vi "parse_package.vi"(8 "error in (no error)":errorcluster, 10 "Raw Package without Header":string, 11 "OXY_SCPI Reseource In":refnum<visa-resource-name>) -> (0 "error out":errorcluster, 2 "DataAllChannels":T1[](array[typedef]), 3 "OXY_SCPI Reseource Out":refnum<visa-resource-name>)   [LabVIEW 2020, in "OXYGEN_Datastream.lvlib"]
uses:
  OXYGEN_Datastream.lvlib
  TypeDefs/DataPoint_Variant.ctl
  TypeDefs/FGV_enum_GeneralInfo.ctl
panel:
  out "error pckg info":u32
  out "Error pckg size":u32
  out "error remeining string":string
  out "error pckg info":string
  out "Error pckg size":string
  out "substring before match":string
  out "packages array":string[](array[string])
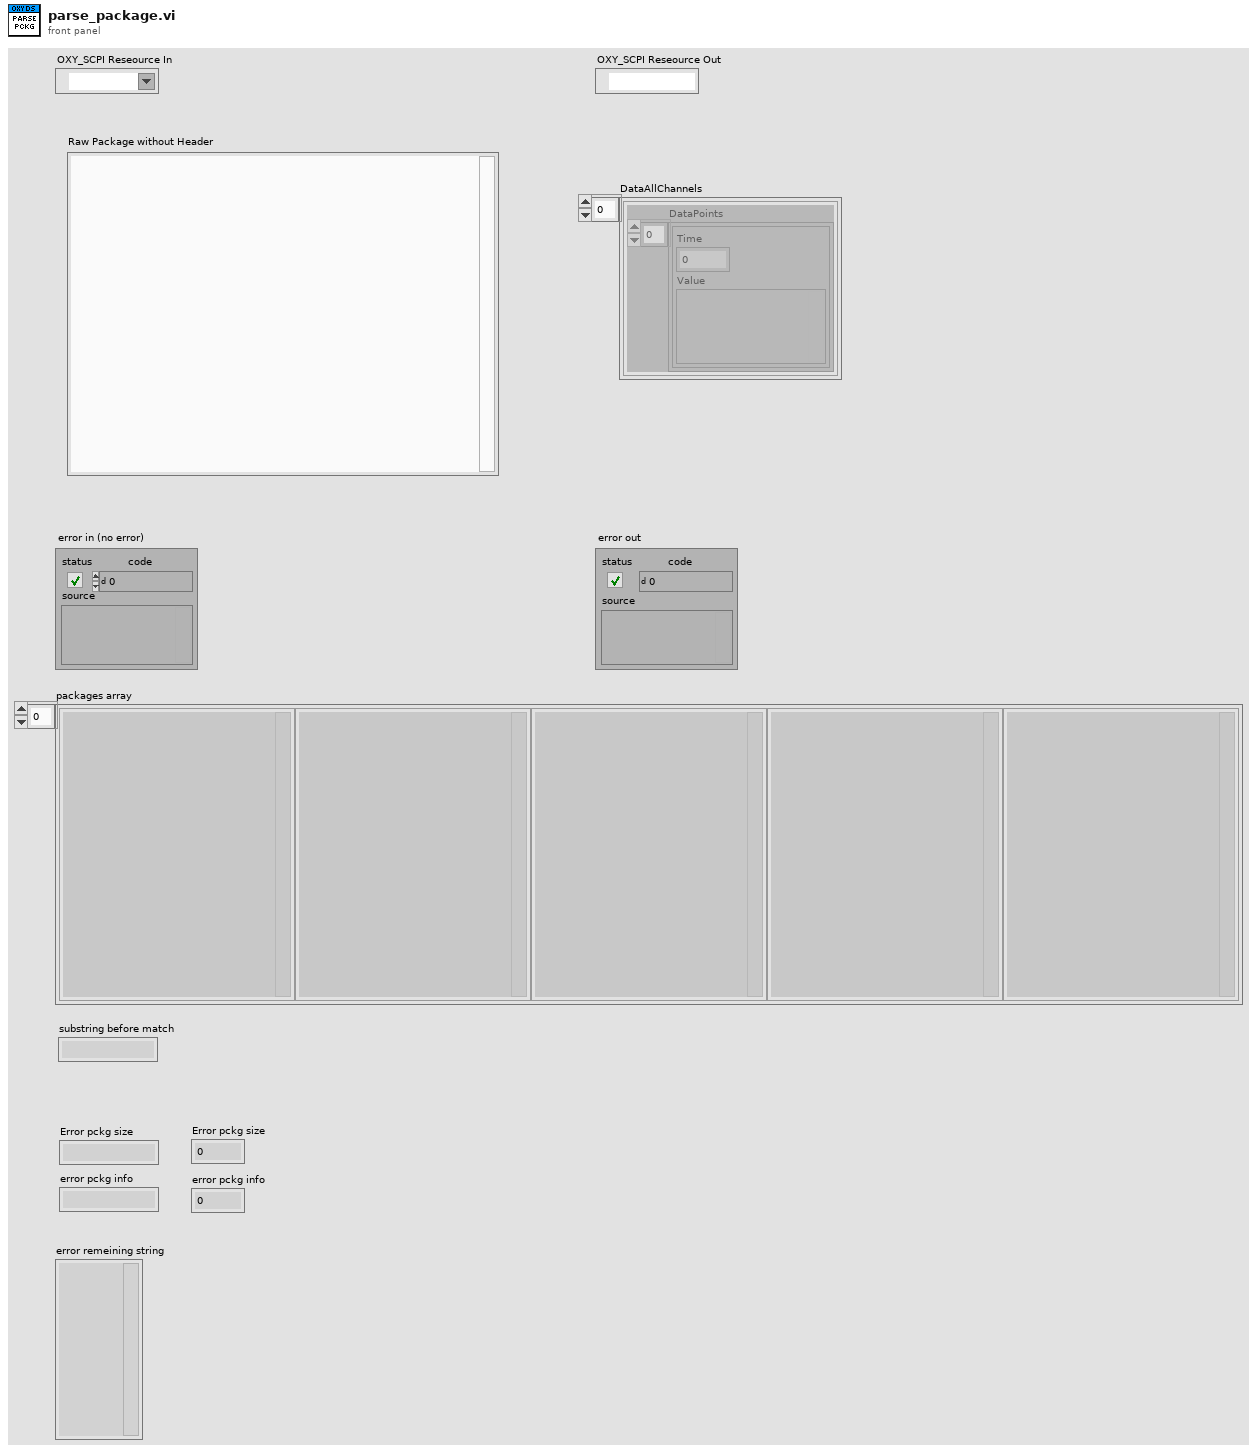
[diagram p1: front panel]
types:
  T1 = typedef "OXYGEN_Datastream.lvlib/DataPoint_Variant.ctl" = cluster{"DataPoints":cluster{"Time":dbl, "Value":variant}[]}
  T2 = typedef "OXYGEN_Datastream.lvlib/FGV_enum_GeneralInfo.ctl" = enum16{"Set_AcqInfo", "Set_ChInfo", "Get"}
  T3 = enum16{"big-endian, network order", "native, host order", "little-endian"}
  T4 = typedef "OXYGEN_Datastream.lvlib/ChannelInfo.ctl" = cluster{"Name":string, "Unit":string, "Scaling":T5}
  T5 = typedef "OXYGEN_Datastream.lvlib/ChannelInfo_Scaling.ctl" = cluster{"factor":dbl, "offset":dbl}
  T6 = typedef "OXYGEN_Datastream.lvlib/AcqInfo_AcquisitionStart.ctl" = cluster{"ISO8061":string, "nanoseconds":T7}
  T7 = typedef "OXYGEN_Datastream.lvlib/AcqInfo_AcquisitionStart_nanoseconds.ctl" = cluster{"utc_offset_seconds":i64, "timestamp_nanoseconds":i64}
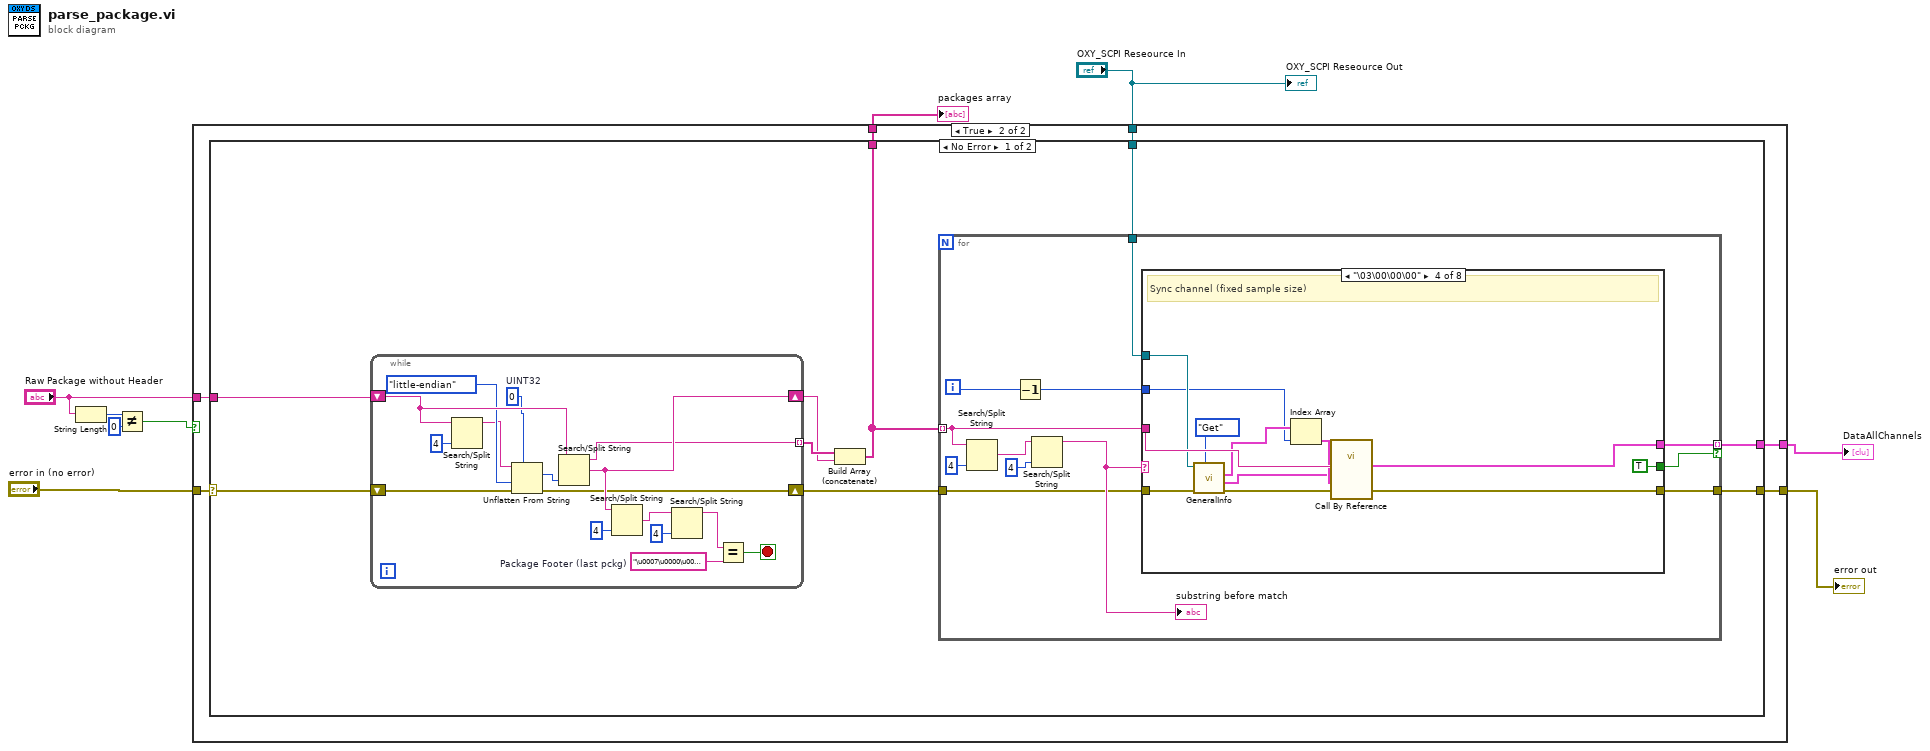
[diagram p0: block diagram]
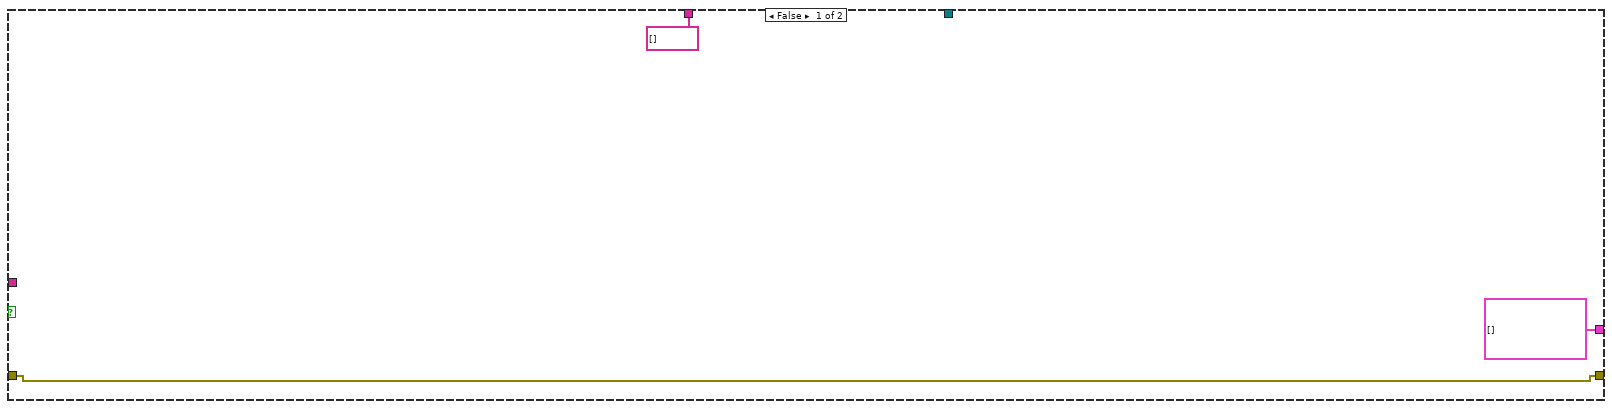
[diagram p2: hidden frame]
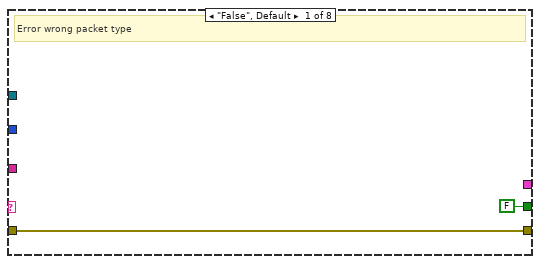
[diagram p3: hidden frame]
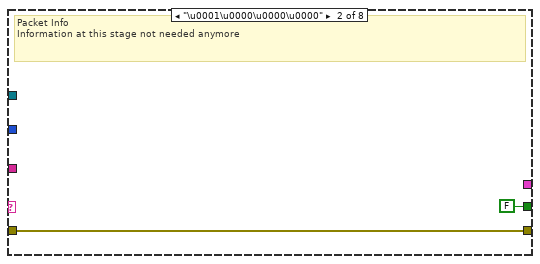
[diagram p4: hidden frame]
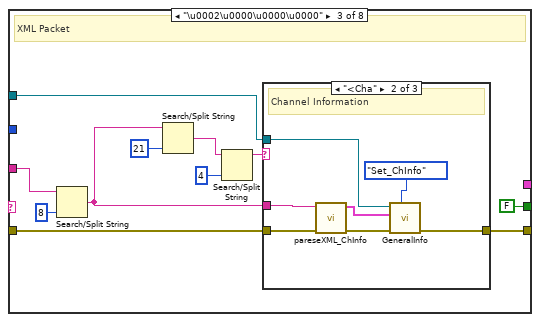
[diagram p5: hidden frame]
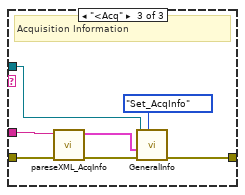
[diagram p7: hidden frame]
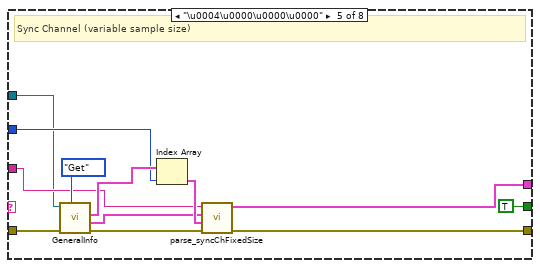
[diagram p8: hidden frame]
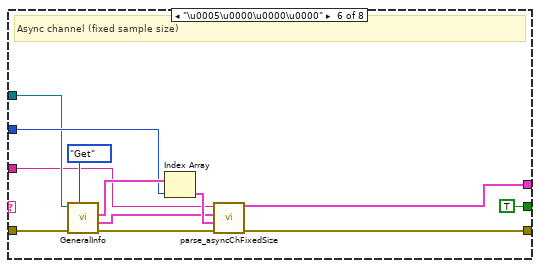
[diagram p9: hidden frame]
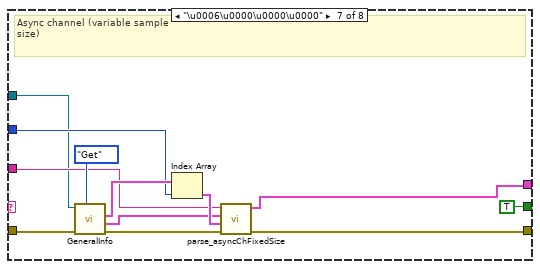
[diagram p10: hidden frame]
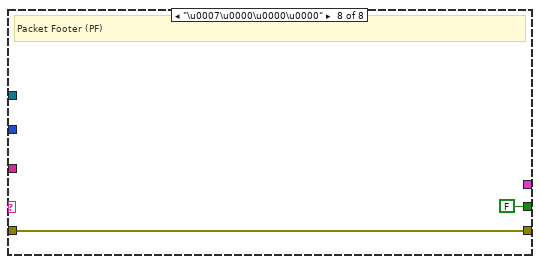
[diagram p11: hidden frame]
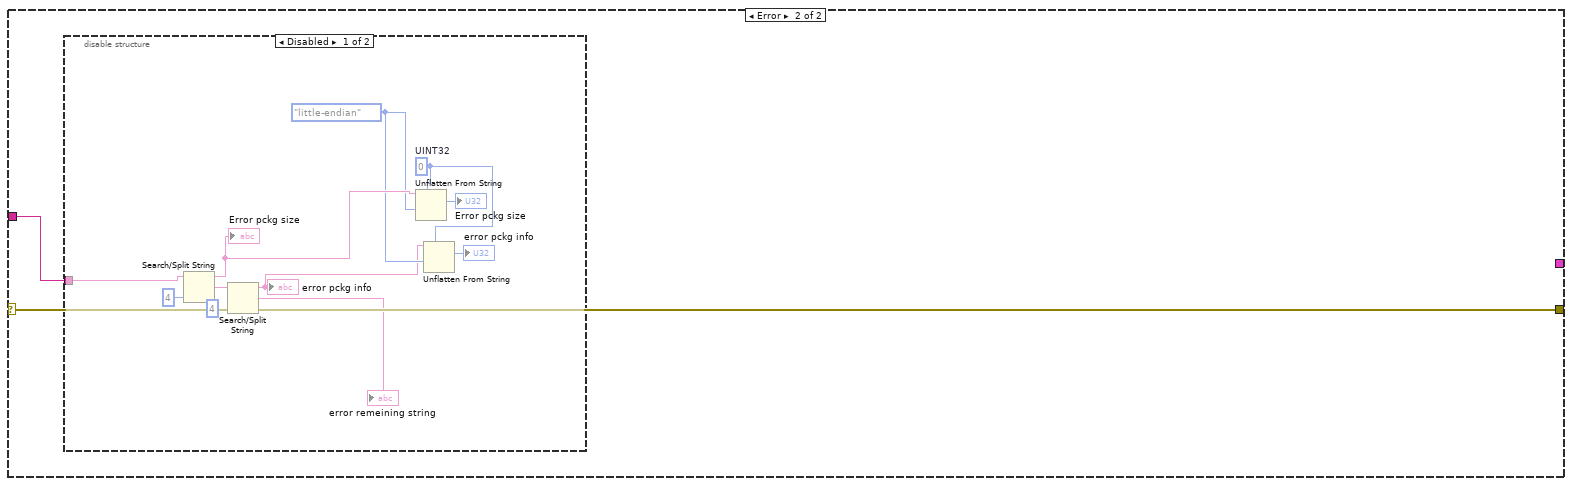
[diagram p12: hidden frame]
diagram:
  n1 = String Length(string="Raw Package without Header") -> (length=w5:i32)
  n2 = Not Equal?(x=w5, y=0) -> (x != y?=w2:bool)
  n3 = case shown="True" w2 {
    tunnel: "Raw Package without Header" -> [_ w18]
    tunnel: [string[] [] w17] -> w9
    tunnel: "OXY_SCPI Reseource In" -> [_ w16]
    tunnel: "error in (no error)" -> [w10 w15]
    tunnel: [w10 w14] -> w6
    tunnel: [T1[] [] w13] -> w1
    frame False {
    }
    frame True {
      n4 = case shown="No Error" w15 {
        selector: w15 -> [w21 w137]
        tunnel: w18 -> [w27 w136]
        tunnel: [w24 _] -> w17
        tunnel: w16 -> [w23 _]
        tunnel: [w19 w137] -> w14
        tunnel: [w22 _] -> w13
        frame No Error {
          n5 = while {
            shift-right: [w127] -> w25
            shift-left: w27 -> [w134]
            tunnel: [w122] -> w26 mode=indexing
            shift-right: [w120] -> w20
            shift-left: w21 -> [w121]
            stop <- w123 stop-if-true
            w126 = "\u0007\u0000\u0000\u0000"  # Package Footer (last pckg)
            w132 = u32 0  # UINT32
            n6 = Search/Split String(string=w134, offset (0)=4) -> (substring before match=w125:string)  [unwired: 1 in, 2 out]
            n7 = Unflatten From String(type=w132, binary string=w125, byte order (0:big-endian, network order)=T3."little-endian", error in (no error)=w121) -> (value=w131:u32, error out=w120:errorcluster)  [unwired: 1 in, 1 out]
            n8 = Search/Split String(string=w134, offset (0)=w131) -> (substring before match=w122:string, match + rest of string=w127:string)  [unwired: 1 in, 1 out]
            n9 = Search/Split String(string=w127, offset (0)=4) -> (match + rest of string=w128:string)  [unwired: 1 in, 2 out]
            n10 = Search/Split String(string=w128, offset (0)=4) -> (substring before match=w124:string)  [unwired: 1 in, 2 out]
            n11 = Equal?(x=w124, y=w126) -> (x = y?=w123:bool)
          }
          n12 = Build Array (concatenate)(w26, w25) -> (w24:string[])
          n13 = for {
            tunnel: w24 -> [w35] mode=indexing
            tunnel: w23 -> [w34]
            tunnel: [w31] -> w22 mode=indexing if=w28
            tunnel: w20 -> [w30]
            tunnel: [w29] -> w19
            i -> [w33]
            n14 = Search/Split String(string=w35, offset (0)=4) -> (match + rest of string=w39:string)  [unwired: 1 in, 2 out]
            n15 = Decrement(x=w33) -> (x-1=w32:i32)
            n16 = Search/Split String(string=w39, offset (0)=4) -> (substring before match=w36:string)  [unwired: 1 in, 2 out]
            "substring before match" <- w36
            n17 = case shown="\"\\03\\00\\00\\00\"" w36 {
              tunnel: w35 -> [_ _ w51 w81 w87 w98 w111 _]
              tunnel: w34 -> [_ _ w47 w78 w84 w102 w109 _]
              tunnel: w32 -> [_ _ _ w75 w86 w103 w110 _]
              tunnel: [_ _ _ w71 w83 w95 w107 _] -> w31
              tunnel: [FALSE FALSE FALSE TRUE TRUE TRUE TRUE FALSE] -> w28
              tunnel: w30 -> [w41 w43 w46 w72 w88 w96 w112 w119]
              tunnel: [w41 w43 w45 w70 w82 w94 w106 w119] -> w29
              frame "False", Default {
                # "Error wrong packet type"
              }
              frame "\u0001\u0000\u0000\u0000" {
                # "Packet Info\nInformation at this stage not needed anymore"
              }
              frame "\u0002\u0000\u0000\u0000" {
                # "XML Packet"
                n18 = Search/Split String(string=w51, offset (0)=8) -> (match + rest of string=w49:string)  [unwired: 1 in, 2 out]
                n19 = Search/Split String(string=w49, offset (0)=21) -> (match + rest of string=w48:string)  [unwired: 1 in, 2 out]
                n20 = Search/Split String(string=w48, offset (0)=4) -> (substring before match=w52:string)  [unwired: 1 in, 2 out]
                n21 = case shown="\"<Cha\"" w52 {
                  tunnel: w49 -> [_ w62 w67]
                  tunnel: w47 -> [_ w58 w65]
                  tunnel: w46 -> [w55 w57 w64]
                  tunnel: [w55 w56 w63] -> w45
                  frame Default {
                    # "unsupported XML format"
                  }
                  frame "<Cha" {
                    # "Channel Information"
                    n22 = call "pareseXML_ChInfo.vi"("error in (no error)"=w57, "Raw Package without Header"=w62) -> ("error out"=w59:errorcluster, "ChannelInfo"=w61:T4[])  [unwired: 8 in]
                    n23 = call "GeneralInfo.vi"("Mode"=FGV_enum_GeneralInfo."Set_ChInfo", "error in (no error)"=w59, "ChannelInfo in"=w61, "OXY_SCPI Reseource In"=w58) -> ("error out"=w56:errorcluster)  [unwired: 5 in, 2 out]
                  }
                  frame "<Acq" {
                    # "Acquisition Information"
                    n24 = call "pareseXML_AcqInfo.vi"("error in (no error)"=w64, "Raw Package without Header"=w67) -> ("error out"=w69:errorcluster, "AcquisitionInfo"=w66:T6)  [unwired: 8 in]
                    n25 = call "GeneralInfo.vi"("Mode"=FGV_enum_GeneralInfo."Set_AcqInfo", "error in (no error)"=w69, "AcquisitionStart"=w66, "OXY_SCPI Reseource In"=w65) -> ("error out"=w63:errorcluster)  [unwired: 5 in, 2 out]
                  }
                }
              }
              frame "\u0003\u0000\u0000\u0000" {
                # "Sync channel (fixed sample size)"
                n26 = call "GeneralInfo.vi"("Mode"=FGV_enum_GeneralInfo."Get", "error in (no error)"=w72, "OXY_SCPI Reseource In"=w78) -> ("error out"=w80:errorcluster, "AcquisitionStart out"=w73:T6, "ChannelInfo out"=w77:T4[])  [unwired: 6 in]
                n27 = Index Array(array=w77, index=w75) -> (element=w76:T4)
                n28 = call-by-ref "?"("error in (no error)"=w80, "ChannelInfo"=w76, "AcquisitionStart"=w73, "Package String"=w81) -> ("error out"=w70:errorcluster, "Data"=w71:T1)  [unwired: 6 in, 4 out]
              }
              frame "\u0004\u0000\u0000\u0000" {
                # "Sync Channel (variable sample size)"
                n29 = call "GeneralInfo.vi"("Mode"=FGV_enum_GeneralInfo."Get", "error in (no error)"=w88, "OXY_SCPI Reseource In"=w84) -> ("error out"=w93:errorcluster, "AcquisitionStart out"=w89:T6, "ChannelInfo out"=w91:T4[])  [unwired: 6 in]
                n30 = Index Array(array=w91, index=w86) -> (element=w90:T4)
                n31 = call "parse_syncChFixedSize.vi"("error in (no error)"=w93, "ChannelInfo"=w90, "AcquisitionStart"=w89, "Package String"=w87) -> ("error out"=w82:errorcluster, "Data"=w83:T1)  [unwired: 4 in, 2 out]
              }
              frame "\u0005\u0000\u0000\u0000" {
                # "Async channel (fixed sample size)"
                n32 = call "GeneralInfo.vi"("Mode"=FGV_enum_GeneralInfo."Get", "error in (no error)"=w96, "OXY_SCPI Reseource In"=w102) -> ("error out"=w101:errorcluster, "AcquisitionStart out"=w99:T6, "ChannelInfo out"=w104:T4[])  [unwired: 6 in]
                n33 = Index Array(array=w104, index=w103) -> (element=w100:T4)
                n34 = call "parse_asyncChFixedSize.vi"("error in (no error)"=w101, "ChannelInfo"=w100, "AcquisitionStart"=w99, "Package String"=w98) -> ("error out"=w94:errorcluster, "Data"=w95:T1)  [unwired: 5 in, 1 out]
              }
              frame "\u0006\u0000\u0000\u0000" {
                # "Async channel (variable sample\nsize)"
                n35 = call "GeneralInfo.vi"("Mode"=FGV_enum_GeneralInfo."Get", "error in (no error)"=w112, "OXY_SCPI Reseource In"=w109) -> ("error out"=w115:errorcluster, "AcquisitionStart out"=w113:T6, "ChannelInfo out"=w116:T4[])  [unwired: 6 in]
                n36 = Index Array(array=w116, index=w110) -> (element=w114:T4)
                n37 = call "parse_asyncChFixedSize.vi"("error in (no error)"=w115, "ChannelInfo"=w114, "AcquisitionStart"=w113, "Package String"=w111) -> ("error out"=w106:errorcluster, "Data"=w107:T1)  [unwired: 5 in, 1 out]
              }
              frame "\u0007\u0000\u0000\u0000" {
                # "Packet Footer (PF)"
              }
            }
          }
        }
        frame Error {
          n38 = disable-structure shown="Disabled" {
            disable-tunnel: w136 -> [w145 _]
            frame Disabled {
              w140 = u32 0  # UINT32
              w139 = T3."little-endian" ("byte order (0:big-endian, network order)")
              n39 = Search/Split String(string=w145, offset (0)=4) -> (substring before match=w143:string, match + rest of string=w148:string)  [unwired: 1 in, 1 out]
              "Error pckg size" <- w143
              n40 = Search/Split String(string=w148, offset (0)=4) -> (substring before match=w138:string, match + rest of string=→"error remeining string":string)  [unwired: 1 in, 1 out]
              "error pckg info" <- w138
              n41 = Unflatten From String(type=w140, binary string=w143, byte order (0:big-endian, network order)=w139) -> (value=→"Error pckg size":u32)  [unwired: 2 in, 2 out]
              n42 = Unflatten From String(type=w140, binary string=w138, byte order (0:big-endian, network order)=w139) -> (value=→"error pckg info":u32)  [unwired: 2 in, 2 out]
            }
            frame Enabled {
            }
          }
        }
      }
    }
  }
  "error out" <- w6
  "packages array" <- w9
  "DataAllChannels" <- w1
  "OXY_SCPI Reseource Out" <- "OXY_SCPI Reseource In"
